vi "Get Integrated Area.vi"(8 "error in":errorcluster, 9 "fmod":sgl, 10 "p":i32=1, 11 "PAS Cell Data in":refnum<class "PAS Cell Data.lvclass">) -> (0 "error out":errorcluster, 3 "PAS Cell Data out":refnum<class "PAS Cell Data.lvclass">)   [LabVIEW 2016, in "PAS Library.lvlib" / "PAS Cell Data.lvclass"]
doc: "This VI takes an input frequency signal and 1) sets a noise threshold (the value below which the spectrum resembles white noise) , 2) sets bounds over which to integrate, 3) finds the integrated area and 4) returns that integrated area with the noise below the threshold level defined by <B>P</B> removed."
uses:
  PAS Cell Data.lvclass
  PAS Cell Data.lvclass/PAS Cell Data.ctl
  General/Math Utilities.lvlib
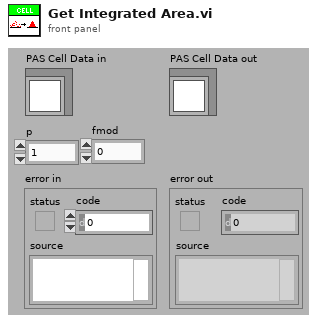
[diagram p1: front panel]
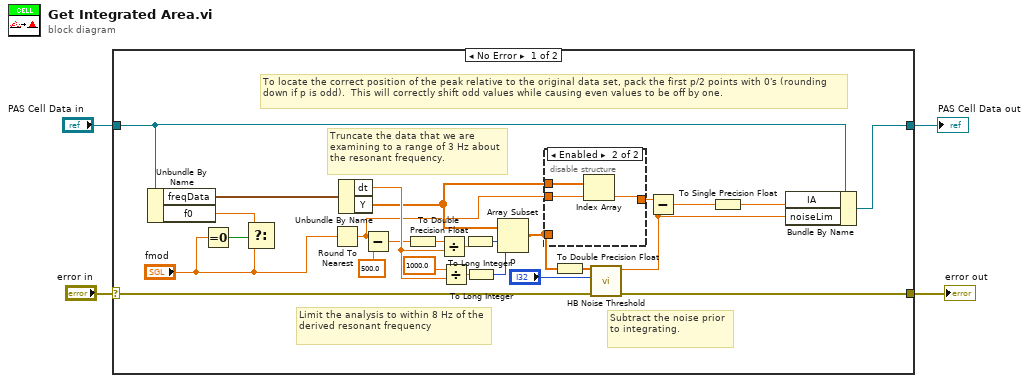
[diagram p0: block diagram]
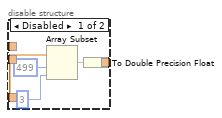
[diagram p2: hidden frame]
diagram:
  n1 = case shown="No Error" "error in" {
    selector: "error in" -> [w26 w40]
    tunnel: [w23 w40] -> w3
    tunnel: [w24 w39] -> w1
    tunnel: "PAS Cell Data in" -> [w12 w39]
    frame No Error {
      # "Truncate the data that we are examining to a range of 3 Hz about the resonant frequency."
      # "To locate the correct position of the peak relative to the original data set, pack the first p/2 points with 0's (rounding down if p is odd).  This will correctly shift odd values while causing even values to be off by one."
      # "Subtract the noise prior to integrating."
      # "Limit the analysis to within 8 Hz of the derived resonant frequency"
      n2 = Unbundle By Name(w12) -> ("freqData"=w27:waveform(sgl), "f0"=w5:sgl)
      n3 = Equal To 0?(x="fmod") -> (x = 0?=w6:bool)
      n4 = Select(t=w5, s=w6, f="fmod") -> ()  [unwired: 1 out]
      n5 = Round To Nearest(number="fmod") -> (nearest integer value=w9:sgl)
      n6 = Unbundle By Name(w27) -> ("dt"=w25:dbl, "Y"=w10:sgl[])
      n7 = Subtract(x=w9, y=sgl 500.0) -> (x-y=w16:sgl)
      n8 = To Double Precision Float(number=w16) -> (double precision float=w17:dbl)
      n9 = Divide(x=w17, y=w25) -> (x/y=w20:dbl)
      n10 = Divide(x=1000.0, y=w25) -> (x/y=w18:dbl)
      n11 = To Long Integer(number=w20) -> (32bit integer=w21:i32)
      n12 = To Long Integer(number=w18) -> (32bit integer=w19:i32)
      n13 = Array Subset(array=w10, index=w21, length=w19) -> (w15:sgl[])
      n14 = disable-structure shown="Enabled" {
        disable-tunnel: w15 -> [w33 _]
        disable-tunnel: [w32 w36] -> w13
        disable-tunnel: w10 -> [_ w38]
        disable-tunnel: w9 -> [_ w37]
        frame Disabled {
          n15 = Array Subset(array=w33, index=499, length=3) -> (w31:sgl[])
          n16 = To Double Precision Float(number=w31) -> (double precision float=w32:dbl[])
        }
        frame Enabled {
          n17 = Index Array(array=w38, index=w37) -> (element=w36:sgl)
        }
      }
      n18 = To Double Precision Float(number=w15) -> (double precision float=w14:dbl[])
      n19 = call "HB Noise Threshold.vi"("Error In"=w26, "p"="p", "Y"=w14) -> ("Error Out"=w23:errorcluster, "P"=w22:dbl)  [unwired: 7 out]
      n20 = Subtract(x=w13, y=w22) -> (x-y=w8:dbl)
      n21 = To Single Precision Float(number=w8) -> (single precision float=w11:sgl)
      n22 = Bundle By Name(cluster=w12, "IA"=w11, "noiseLim"=w22) -> (w24:refnum<class "PAS Cell Data.lvclass">)
    }
    frame Error {
    }
  }
  "error out" <- w3
  "PAS Cell Data out" <- w1
